vi "GlobalSetGetTriggerForPointMeasurement.vi"() -> ()   [LabVIEW 2011]
panel:
  in  "PulseSequenzelength":i32
  in  "Initial delay":dbl
  in  "Duty Cycle":dbl
  in  "Frequency":dbl
  in  "Nr.Pulses":i32
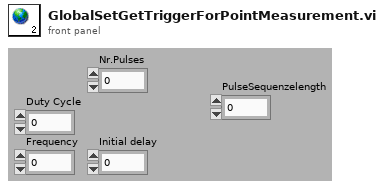
[diagram p1: front panel]
diagram:
